vi "Image Processing_Feng.vi"(0 "File Path":path=path "C:/General AFM lithography program/Sample.ibw", 1 "Lithography Information":T2(array[cluster])=array7x3944[27608 elements], 2 "Crop?":bool, 3 "Crop Data":T3, 4 "Angle (degrees)":dbl, 5 "error in (no error)":errorcluster, 6 "Size":cluster{"Width":dbl, "Height":dbl}={"Width"=40.0, "Height"=40.0}, 7 "Page":i32=1, 8 "Interested image data min":dbl(slide) min=0.0 max=100.0 scale=0.0..100.0, 10 "Interested image data max":dbl(slide)=100.0 min=0.0 max=100.0 scale=0.0..100.0, 11 "Resolution":i32=1024) -> (14 "Image Out":T4(plugin-control), 15 "Offset":T1={"X Offset (µm)"=-1.2812, "Y Offset (µm)"=5.2969}, 16 "Sample Size":cluster{"Width (µm)":dbl, "Height (µm)":dbl}={"Width (µm)"=40.0, "Height (µm)"=40.0}, 19 "error out":errorcluster)   [LabVIEW 2013]
uses:
  <vilib>/vision/NI_Vision_Development_Module.lvlib
panel:
  out "Suggested max":dbl
  out "Suggested min":dbl
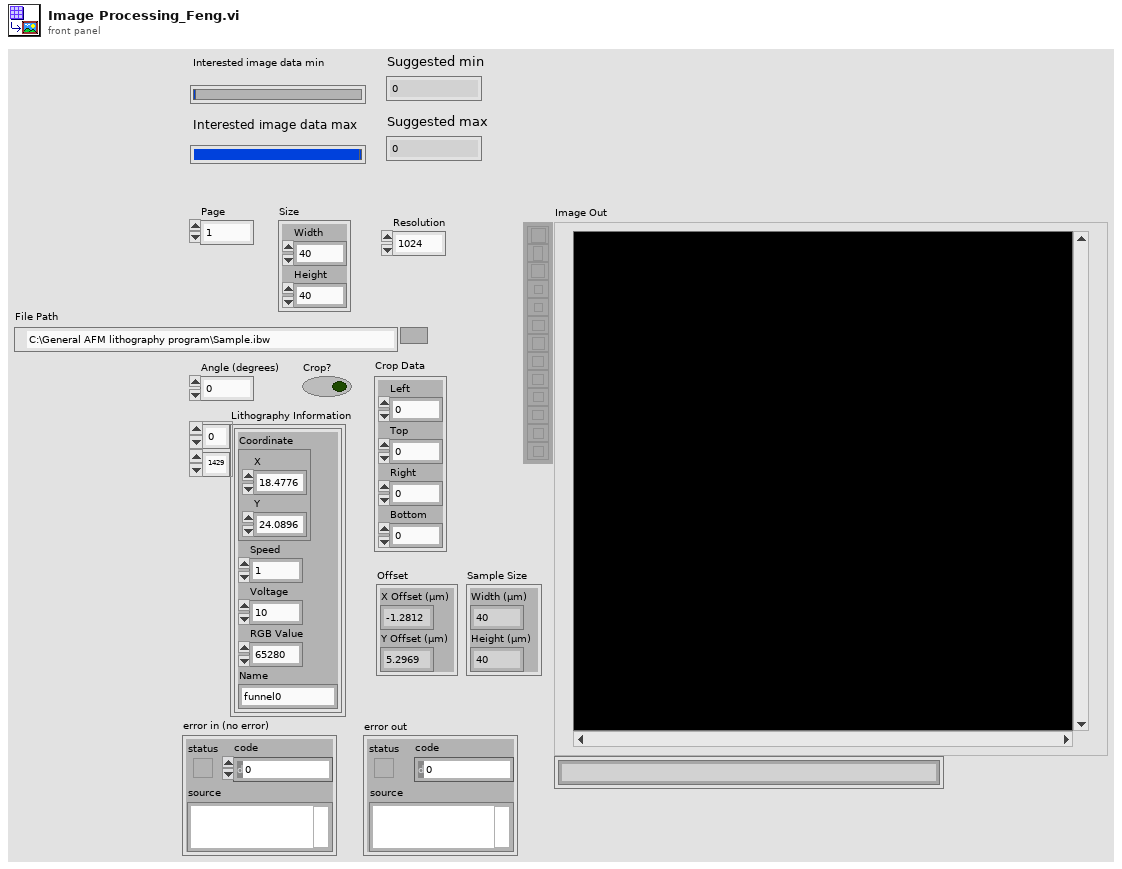
[diagram p1: front panel]
types:
  T1 = cluster{"X Offset (µm)":dbl, "Y Offset (µm)":dbl}
  T2 = cluster{"Coordinate":cluster{"X":dbl, "Y":dbl}, "Speed":dbl, "Voltage":dbl, "RGB Value":i32, "Name":string}[][]
  T3 = cluster{"Left":dbl, "Top":dbl, "Right":dbl, "Bottom":dbl}
  T4 = typedef "IMAQ Image.ctl" = refnum<image>
  T5 = typedef "Image Type" = u32
  T6 = cluster{"Coordinate":cluster{"X":dbl, "Y":dbl}, "Speed":dbl, "Voltage":dbl, "RGB Value":i32, "Name":string}
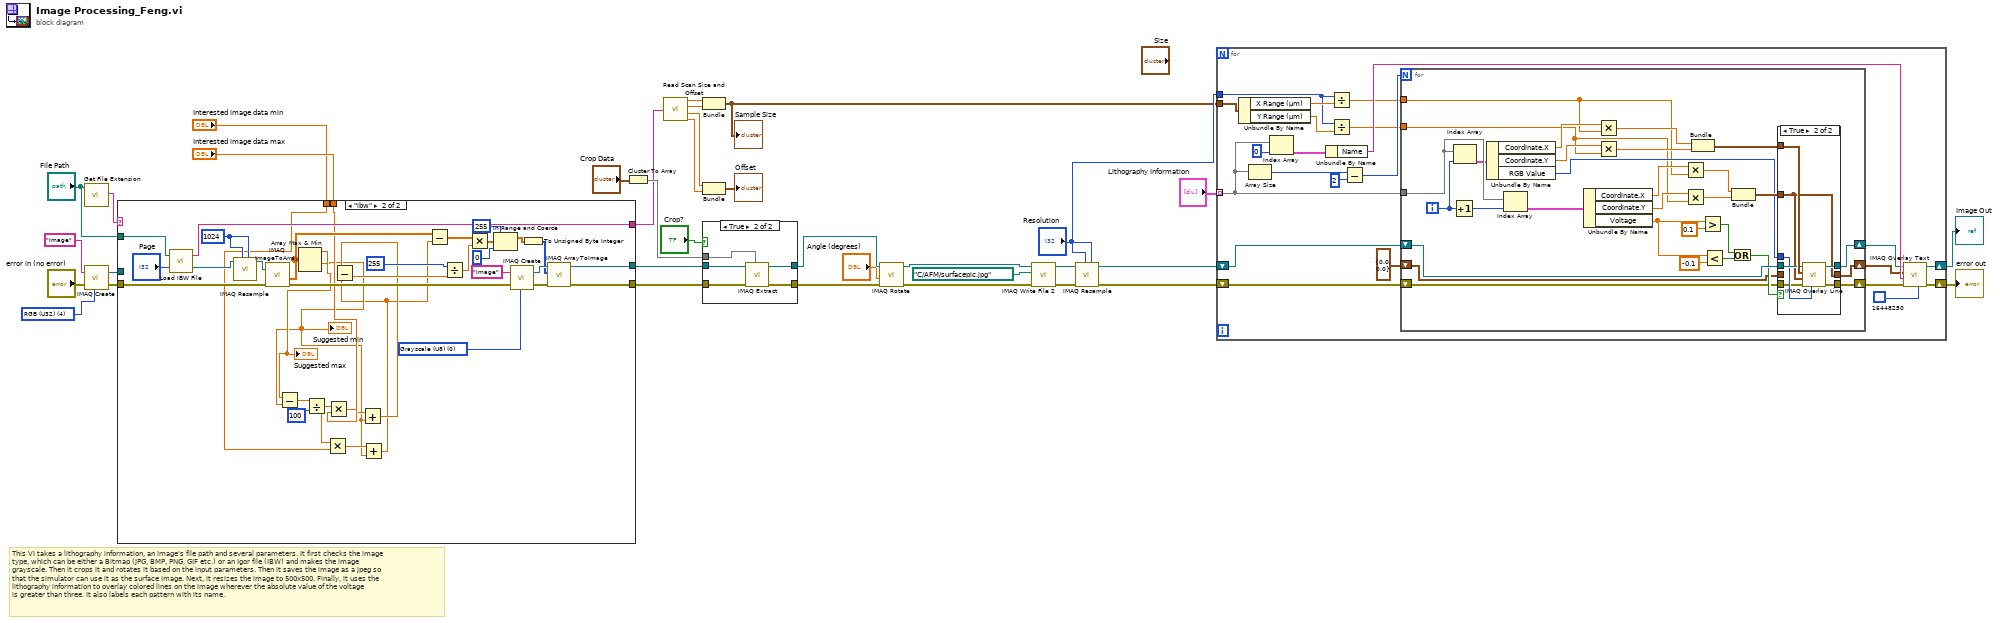
[diagram p0: block diagram]
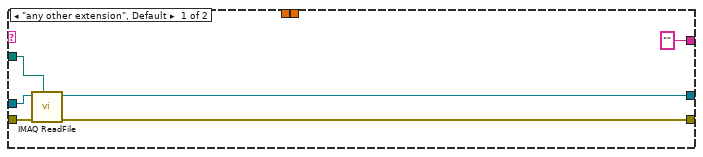
[diagram p2: hidden frame]
diagram:
  w34 = T5 4 items=["Grayscale (U8)", "Grayscale (I16)", "Grayscale (SGL)", "Complex (CSG)", "RGB (U32)", "HSL (U32)", "RGB (U64)", "Grayscale (U16)"] ("Image Type")
  # "This VI takes a lithography information, an image's file path and several parameters. It first checks the image \ntype, which can be either a Bitmap (JPG, BMP, PNG, GIF etc.) or an Igor file (IBW) and makes the image \ngrayscale. Then it crops it and rotates it based on the input parameters. Then it saves the image as a jpeg so \nthat the simulator can use it as the surface image. Next, it resizes the image to 500x500. Finally, it uses the \nlithography information to overlay colored lines on the image wherever the absolute value of the voltage \nis greater than three. It also labels each pattern with its name."
  n1 = call <vilib>:"Get File Extension.vi"("file"="File Path") -> ("lowercase file extension"=w21:string)  [unwired: 7 in, 3 out]
  n2 = call "IMAQ Create"("Image Name"="Image", "Image Type"=w34, "error in (no error)"="error in (no error)") -> ("New Image"=w33:T4, "error out"=w32:errorcluster)  [unwired: 2 in]
  n3 = case shown="\"ibw\"" w21 {
    tunnel: w33 -> [w41 _]
    tunnel: w32 -> [w40 w74]
    tunnel: [w39 w67] -> w31
    tunnel: [w38 w66] -> w30
    tunnel: "File Path" -> [w37 w76]
    tunnel: ["" ("Wave Note") w57] -> w10
    tunnel: "Interested image data max" -> [_ w49]
    tunnel: "Interested image data min" -> [_ w45]
    frame "any other extension", Default {
      n4 = call "IMAQ ReadFile"("File Path"=w37, "error in (no error)"=w40, "Image"=w41) -> ("error out"=w38:errorcluster, "Image Out"=w39:T4)  [unwired: 4 in, 3 out]
    }
    frame "ibw" {
      w64 = 1024 ("Y Resolution")
      w71 = T5 0 items=["Grayscale (U8)", "Grayscale (I16)", "Grayscale (SGL)", "Complex (CSG)", "RGB (U32)", "HSL (U32)", "RGB (U64)", "Grayscale (U16)"] ("Image Type")
      n5 = call "Load IBW File.vi"("Page"="Page", "file path (dialog if empty)"=w76) -> ("Image"=w63:T4, "Wave Note"=w57:string)
      n6 = call "IMAQ Resample"("X Resolution"=w64, "Y Resolution"=w64, "Image Src"=w63) -> ("Image Dst Out"=w62:T4)  [unwired: 7 in, 1 out]
      n7 = call "IMAQ ImageToArray"("error in (no error)"=w74, "Image"=w62) -> ("Image Pixels (Float)"=w73:sgl[][], "error out"=w68:errorcluster)  [unwired: 2 in, 3 out]
      n8 = Array Max & Min(array=w73) -> (max value=w52:sgl, min value=w43:sgl)  [unwired: 2 out]
      "Suggested min" <- w43
      "Suggested max" <- w52
      n9 = Subtract(x=w52, y=w43) -> (x-y=w51:sgl)
      n10 = Divide(x=w51, y=100) -> (x/y=w46:sgl)
      n11 = Multiply(x=w46, y=w45) -> (x*y=w44:dbl)
      n12 = Multiply(x=w46, y=w49) -> (x*y=w48:dbl)
      n13 = Add(x=w48, y=w43) -> (x+y=w47:dbl)
      n14 = Add(x=w44, y=w43) -> (x+y=w42:dbl)
      n15 = Subtract(x=w47, y=w42) -> (x-y=w60:dbl)
      n16 = Subtract(x=w73, y=w42) -> (x-y=w61:dbl[][])
      n17 = Divide(x=255, y=w60) -> (x/y=w58:dbl)
      n18 = Multiply(x=w61, y=w58) -> (x*y=w56:dbl[][])
      n19 = In Range and Coerce(upper limit=255, x=w56, lower limit=0) -> (coerced(x)=w53:dbl[][])  [unwired: 1 out]
      n20 = call "IMAQ Create"("Image Name"="Image", "Image Type"=w71, "error in (no error)"=w68) -> ("New Image"=w72:T4, "error out"=w69:errorcluster)  [unwired: 2 in]
      n21 = To Unsigned Byte Integer(number=w53) -> (unsigned 8bit integer=w70:u8[][])
      n22 = call "IMAQ ArrayToImage"("error in (no error)"=w69, "Image Pixels (U8)"=w70, "Image"=w72) -> ("error out"=w66:errorcluster, "Image Out"=w67:T4)  [unwired: 7 in]
    }
  }
  n23 = Cluster To Array(cluster="Crop Data") -> (array=w28:dbl[])
  n24 = call "Read Scan Size and Offset.vi"("Read in the string file"=w10) -> ("X Range (µm)"=w9:dbl, "Y Range (µm)"=w8:dbl, "X Offset (µm)"=w7:dbl, "Y Offset (µm)"=w6:dbl)  [unwired: 4 in]
  n25 = Bundle("X Range (µm)"=w9, "Y Range (µm)"=w8) -> (w3:cluster{"X Range (µm)":dbl, "Y Range (µm)":dbl})  [unwired: 1 in]
  "Sample Size" <- w3
  n26 = Bundle("X Offset (µm)"=w7, "Y Offset (µm)"=w6) -> (→"Offset":T1)  [unwired: 1 in]
  n27 = case shown="True" "Crop?" {
    tunnel: w31 -> [w78 w82]
    tunnel: w30 -> [w77 w81]
    tunnel: w28 -> [_ w83]
    tunnel: [w78 w79] -> w19
    tunnel: [w77 w80] -> w18
    frame False {
    }
    frame True {
      n28 = call "IMAQ Extract"("Optional Rectangle"=w83, "error in (no error)"=w81, "Image Src"=w82) -> ("error out"=w80:errorcluster, "Image Dst Out"=w79:T4)  [unwired: 7 in]
    }
  }
  n29 = call "IMAQ Rotate"("error in (no error)"=w18, "Angle (degrees)"="Angle (degrees)", "Image Src"=w19) -> ("error out"=w15:errorcluster, "Image Dst Out"=w16:T4)  [unwired: 7 in]
  n30 = call-poly "IMAQ Write File 2"("error in (no error)"=w15, "File Path"=path "C:/AFM/surfacepic.jpg", "Image"=w16) -> ("error out"=w13:errorcluster, "Image Out (duplicate)"=w14:T4)  [unwired: 7 in]
  n31 = call "IMAQ Resample"("X Resolution"="Resolution", "Y Resolution"="Resolution", "error in (no error)"=w13, "Image Src"=w14) -> ("error out"=w11:errorcluster, "Image Dst Out"=w12:T4)  [unwired: 6 in]
  n32 = for {
    tunnel: "Lithography Information" -> [w92] mode=indexing
    shift-right: [w94] -> w23
    shift-left: w12 -> [w100]
    shift-right: [w96] -> w26
    shift-left: w11 -> [w102]
    tunnel: "Resolution" -> [w85]
    tunnel: w3 -> [w84]
    n33 = Unbundle By Name(w84) -> ("X Range (µm)"=w87:dbl, "Y Range (µm)"=w86:dbl)
    n34 = Array Size(array=w92) -> (size(s)=w105:i32)
    n35 = Index Array(array=w92, index=0) -> (element=w90:T6)
    n36 = Unbundle By Name(w90) -> ("Name"=w99:string)
    n37 = Divide(x=w85, y=w87) -> (x/y=w89:dbl)
    n38 = Divide(x=w85, y=w86) -> (x/y=w88:dbl)
    n39 = Subtract(x=w105, y=2) -> (x-y=w103:i32)
    n40 = for {
      N: w103 -> [_]
      tunnel: w92 -> [w113]
      shift-right: [w121] -> w95
      shift-left: w100 -> [w130]
      shift-right: [w114] -> w97
      shift-left: w102 -> [w115]
      tunnel: w89 -> [w109]
      shift-right: [w108] -> w93
      shift-left: cluster{dbl, dbl} {0.0, 0.0} -> [w107]
      tunnel: w88 -> [w106]
      i -> [w112]
      n41 = Increment(x=w112) -> (x+1=w131:i32)
      n42 = Index Array(array=w113, index=w112) -> (element=w111:T6)
      n43 = Unbundle By Name(w111) -> ("Coordinate.X"=w135:dbl, "Coordinate.Y"=w134:dbl, "RGB Value"=w122:i32)
      n44 = Index Array(array=w113, index=w131) -> (element=w128:T6)
      n45 = Unbundle By Name(w128) -> ("Coordinate.X"=w126:dbl, "Coordinate.Y"=w127:dbl, "Voltage"=w110:dbl)
      n46 = Multiply(x=w135, y=w109) -> (x*y=w133:dbl)
      n47 = Multiply(x=w134, y=w106) -> (x*y=w132:dbl)
      n48 = Multiply(x=w126, y=w109) -> (x*y=w125:dbl)
      n49 = Multiply(x=w127, y=w106) -> (x*y=w124:dbl)
      n50 = Bundle(w133, w132) -> (w129:cluster{dbl, dbl})  [unwired: 1 in]
      n51 = Greater?(x=w110, y=0.1) -> (0:w118:bool)
      n52 = Less?(x=w110, y=-0.1) -> (x < y?=w117:bool)
      n53 = Or(x=w118, y=w117) -> (x .or. y?=w116:bool)
      n54 = Bundle(w125, w124) -> (w123:cluster{dbl, dbl})  [unwired: 1 in]
      n55 = case shown="True" w116 {
        tunnel: w130 -> [w138 w143]
        tunnel: w129 -> [_ w145]
        tunnel: w123 -> [_ w139]
        tunnel: w122 -> [_ w142]
        tunnel: [w138 w144] -> w121
        tunnel: w115 -> [w137 w141]
        tunnel: [w137 w140] -> w114
        tunnel: [w136 w139] -> w108
        tunnel: w107 -> [w136 _]
        frame False {
        }
        frame True {
          n56 = call "IMAQ Overlay Line"("Color"=w142, "error in (no error)"=w141, "End Point"=w139, "Start Point"=w145, "Image"=w143) -> ("error out"=w140:errorcluster, "Image Out"=w144:T4)  [unwired: 5 in]
        }
      }
    }
    n57 = call "IMAQ Overlay Text"("BG Color (Transparent)"=u32 16448250, "error in (no error)"=w97, "String"=w99, "Origin"=w93, "Image"=w95) -> ("error out"=w96:errorcluster, "Image Out"=w94:T4)  [unwired: 5 in]
  }
  "Image Out" <- w23
  "error out" <- w26
